vi "Sampler Signals (A).vi"(0 "IsMeasuring":bool, 1 "EI":refnum<k24>, 5 "Sampler":refnum<k24>, 7 "Signal X":string(combo), 9 "Signal Y":string(combo), 11 "error in":errorcluster) -> (3 "PotentialApplied":dbl, 4 "X":dbl, 6 "Y":dbl, 8 "XY Graph":cluster{"Y":dbl[], "Y":dbl[]}[](graph), 10 "GetSignals":string[](array[string]), 15 "error out":errorcluster)   [LabVIEW 2014]
doc: "Shows the signals from the sampler. The signals can manually selected. Only for Cyclic Voltammetry measurements. (advanced version)"
uses:
  C:/Users/user/Documents/Andre/AutoLAB/Autolab SDK 1.11/EcoChemie.Autolab.Sdk.dll
  EcoChemie.Autolab.Sdk.dll
panel:
  out "Reset":bool
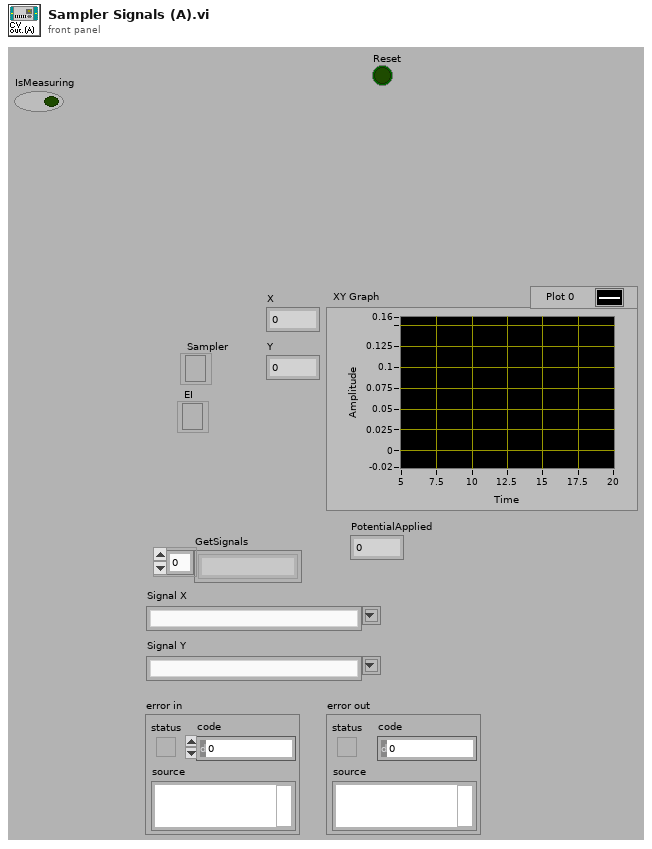
[diagram p1: front panel]
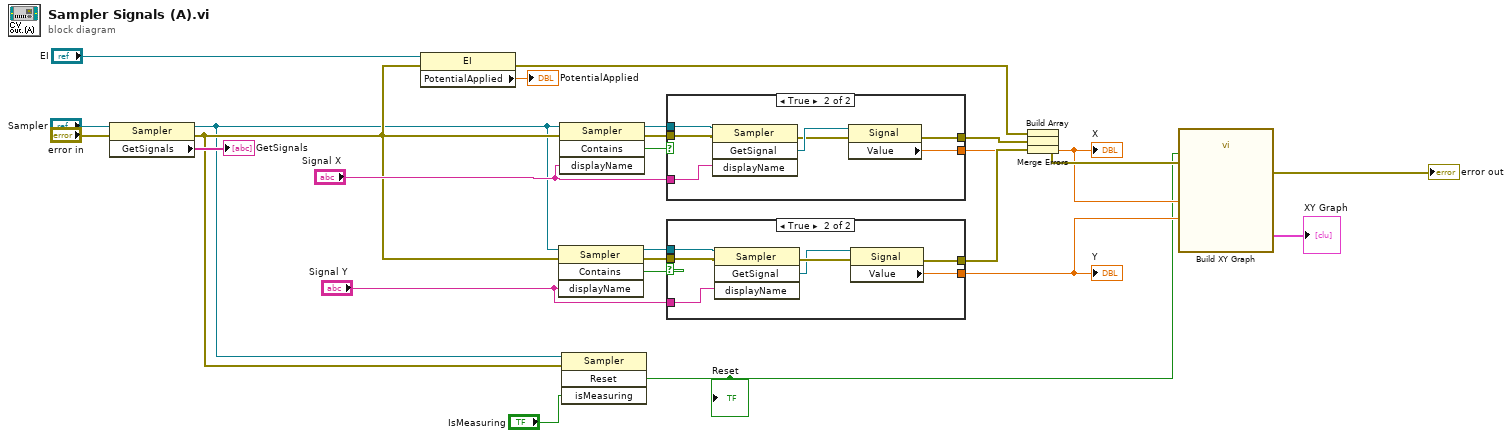
[diagram p0: block diagram]
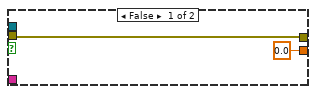
[diagram p2: hidden frame]
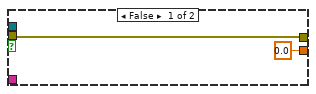
[diagram p3: hidden frame]
diagram:
  n1 = property class="Sampler"(reference="Sampler", error in="error in") -> (reference out=w17:refnum<k24>, error out=w18:errorcluster, "GetSignals"=→"GetSignals":string[])
  n2 = property class="EI"(reference="EI", error in=w18) -> (error out=w7:errorcluster, "PotentialApplied"=→"PotentialApplied":dbl)  [unwired: 1 out]
  n3 = invoke class="Sampler" method="Contains"(reference=w17, error in=w18, "displayName"="Signal Y") -> (reference out=w14:refnum<k24>, error out=w13:errorcluster, "Contains"=w15:bool)  [unwired: 1 in, 1 out]
  n4 = invoke class="Sampler" method="Contains"(reference=w17, error in=w18, "displayName"="Signal X") -> (reference out=w12:refnum<k24>, error out=w11:errorcluster, "Contains"=w16:bool)  [unwired: 1 in, 1 out]
  n5 = invoke class="Sampler" method="Reset"(reference=w17, error in=w18, "isMeasuring"="IsMeasuring") -> ("Reset"=w3:bool)  [unwired: 1 in, 3 out]
  "Reset" <- w3
  n6 = case shown="True" w16 {
    tunnel: [0.0 ("Value") w35] -> w5
    tunnel: "Signal X" -> [_ w34]
    tunnel: w11 -> [w28 w33]
    tunnel: w12 -> [_ w32]
    tunnel: [w28 w31] -> w6
    frame False {
    }
    frame True {
      n7 = invoke class="Sampler" method="GetSignal"(reference=w32, error in=w33, "displayName"=w34) -> (error out=w29:errorcluster, "GetSignal"=w30:refnum<k24>)  [unwired: 1 in, 2 out]
      n8 = property class="Signal"(reference=w30, error in=w29) -> (error out=w31:errorcluster, "Value"=w35:dbl)  [unwired: 1 out]
    }
  }
  "X" <- w5
  n9 = case shown="True" w15 {
    tunnel: "Signal Y" -> [_ w44]
    tunnel: [0.0 ("Value") w43] -> w4
    tunnel: w13 -> [w37 w42]
    tunnel: w14 -> [_ w41]
    tunnel: [w37 w38] -> w10
    frame False {
    }
    frame True {
      n10 = invoke class="Sampler" method="GetSignal"(reference=w41, error in=w42, "displayName"=w44) -> (error out=w40:errorcluster, "GetSignal"=w39:refnum<k24>)  [unwired: 1 in, 2 out]
      n11 = property class="Signal"(reference=w39, error in=w40) -> (error out=w38:errorcluster, "Value"=w43:dbl)  [unwired: 1 out]
    }
  }
  "Y" <- w4
  n12 = Build Array(w7, w6, w10) -> (w1:errorcluster[])
  n13 = Merge Errors(w1) -> (w9:errorcluster)
  n14 = call "Build XY Graph"("error in (no error)"=w9, "Reset"=w3, "Y Input"=w4, "X Input"=w5) -> ("error out"=→"error out":errorcluster, "XY Graph"=→"XY Graph":cluster{"Y":dbl[], "Y":dbl[]}[])  [unwired: 6 in]
